vi "RoomAlert.vi"() -> ()   [LabVIEW 2018, in "Visualization.lvlib" / "VisualizeSensor.lvclass"]
doc: "This VI listens for any measurement data associated with the provided PluginName and displays it to the user for analysis. The display is only suitable for data coming from the RoomAlert Plugin."
uses:
  VisualizeSensor.lvclass
  VisualizeBase/VisualizeBase_class/SubVIs/VisualizationOptions.ctl
  <vilib>/Utility/miscctls.llb/LVRectTypeDef.ctl
  Sensor/SensorShared/clSensorData.ctl
  <vilib>/event_ctls.llb/usereventprio.ctl
  VisualizeBase/VisualizeBase_class/Requests/VisUserEventType.ctl
  <extravilib>/ChannelInstances/Tag-bool/Write With Abort.vi
  <extravilib>/ChannelInstances/Tag-bool/Read With Abort.vi
  <extravilib>/ChannelInstances/Tag-bool/Instantiate.vi
  <extravilib>/ChannelInstances/Tag-bool/EndpointRead.vi
  <vilib>/Utility/error.llb/Error Cluster From Error Code.vi
  <extravilib>/ChannelInstances/Tag-bool/Endpoint.vi
  <vilib>/ErrorRing/Error Ring.xnode
  <userlib>/NIST/NISTErrorLib/NISTErrorLib.lvlib
  VisualizeBase/VisualizeBase_class/VisualizeBase.lvclass
  Sensor/SensorShared/SensorShared.lvlib
  Sensor/SensorModule/SensorModule.lvlib
  <extravilib>/ChannelInstances/Tag-bool.lvlib
  TestClass/Test.lvclass
  StatusAndLog/VisualizeStatus.lvclass
  Sensor/SensorPlugins/SensorPlugins.lvlib
panel:
  in  "btnPause":bool=TRUE
  out "VisualizationProperties":T1={"PauseAtStartup"=TRUE, "LogData"=FALSE, "LaunchInSubPanel"=TRUE, "FPMonitor"=0, "FPWindowBounds"={"Left"=0, "Top"=0, "Right"=0, "Bottom"=0}, "MonitorBounds"={"Left"=0, "Top"=0, "Right"=0, "Bottom"=0}}
  in  "INIFilePath":path
  in  "ModuleID":i32
  in  "Log Data":bool=TRUE
  in  "btnStop":bool
  in  "btnReset":bool
  in  "btnClearTest":bool
  in  "btnStopModule":bool
  out "Chart":waveform(dbl)[](graph)=[{"t0"=timestamp(3657200531.6397257 s since 1904-01-01), "dt"=1.0, "Y"=[46.19]}, {"t0"=timestamp(3657200531.6397257 s since 1904-01-01), "dt"=1.0, "Y"=[2.0]}, {"t0"=timestamp(3657200531.6397257 s since 1904-01-01), "dt"=1.0, "Y"=[60.0]}]
  out "LightTower":T3
  out "ErrorArray":errorcluster[](array[cluster])
  out "Incorrect DataType?":bool
  out "String Results":string="Sensor.RoomAlert1"
  in  "PluginName":string="Sensor.RoomAlert1"
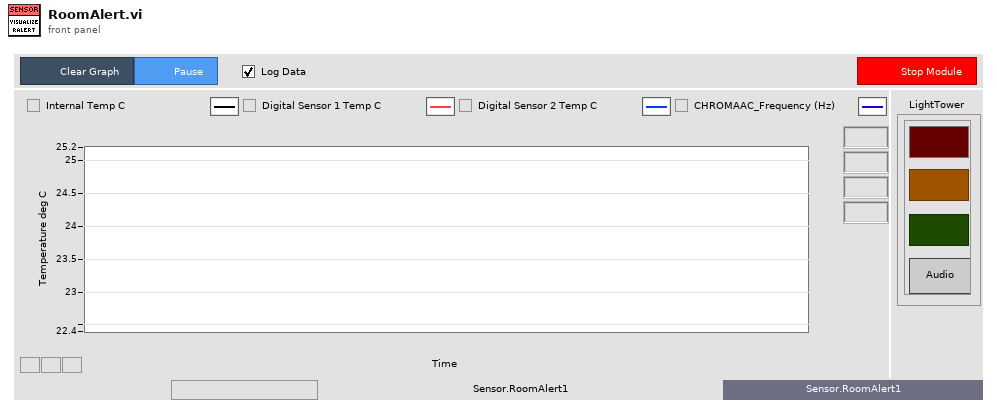
[diagram p1: front panel]
types:
  T1 = typedef "Visualization.lvlib/VisualizeBase.lvclass/VisualizationOptions.ctl" = cluster{"PauseAtStartup":bool, "LogData":bool, "LaunchInSubPanel":bool, "FPMonitor":u16, "FPWindowBounds":T2, "MonitorBounds":cluster{"Left":i16, "Top":i16, "Right":i16, "Bottom":i16}}
  T2 = typedef "LVRectTypeDef.ctl" = cluster{"Left":i16, "Top":i16, "Right":i16, "Bottom":i16}
  T3 = cluster{"Red":bool, "Amber":bool, "Green":bool, "Audio":bool}
  T4 = enum16{"open", "open or create", "create or replace", "create", "open (read-only)"}
  T5 = typedef "Visualization.lvlib/VisualizeBase.lvclass/VisRequestEvents.ctl" = cluster{"StopRequest":refnum<user-event>, "ResetRequest":refnum<user-event>, "FP Pop In or Out":refnum<user-event>}
  T6 = typedef "SensorShared.lvlib/clBroadcastEvents.ctl" = cluster{"DidInit":refnum<user-event>, "StatusUpdate":refnum<user-event>, "ErrorReport":refnum<user-event>, "DidStop":refnum<user-event>, "PathToINI":refnum<user-event>, "SensorReport":refnum<user-event>, "SensorConfig":refnum<user-event>}
  T7 = typedef "SensorShared.lvlib/clSensorData.ctl" = cluster{"SensorType":string, "SensorData":variant}
  T8 = typedef "Visualization.lvlib/VisualizeBase.lvclass/VisUserEventType.ctl" = cluster{"BusIndex":i8, "Data":variant}
  T9 = typedef "usereventprio.ctl" = enum32{"high priority", "normal priority"}
  T10 = cluster{"Red":bool, "Amber":bool, "Green":bool, "Audio":bool}[]
  T11 = typedef "Tag-bool.lvlib/))Channel.ctl" = refnum<queue>
  T12 = typedef "sizeaction.ctl" = enum32{"Minimized", "Maximized", "Resized"}
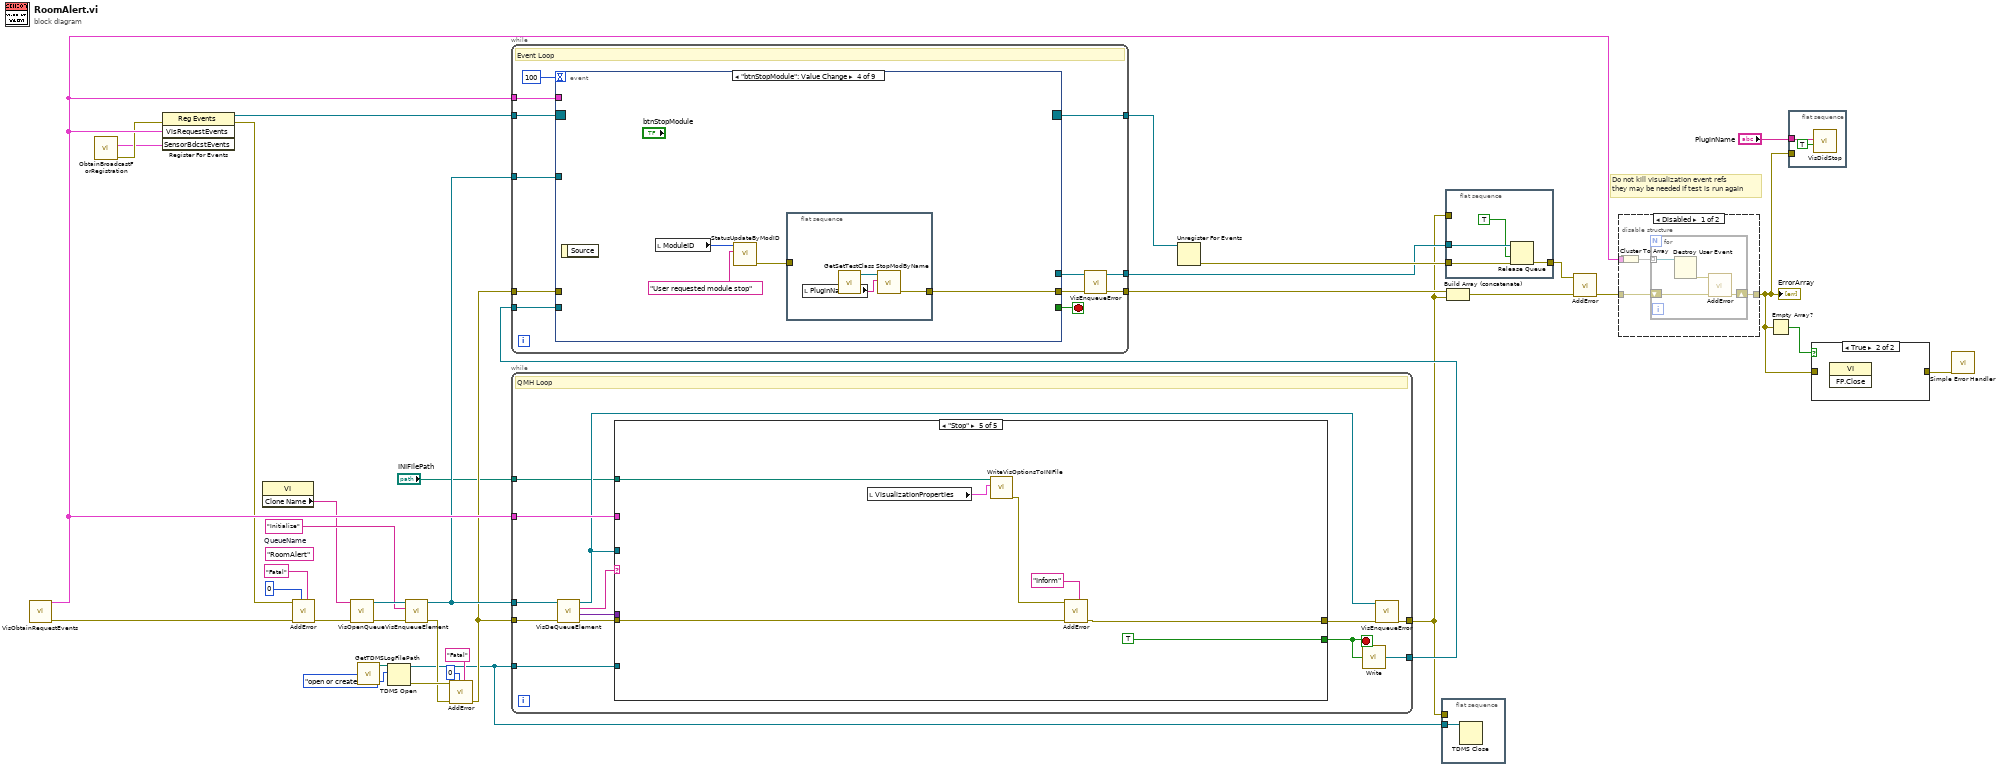
[diagram p0: block diagram]
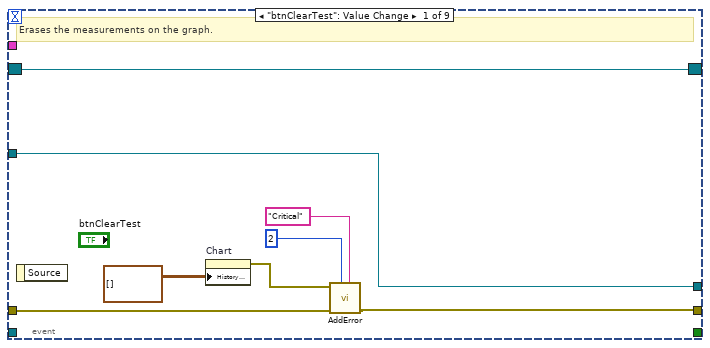
[diagram p3: hidden frame]
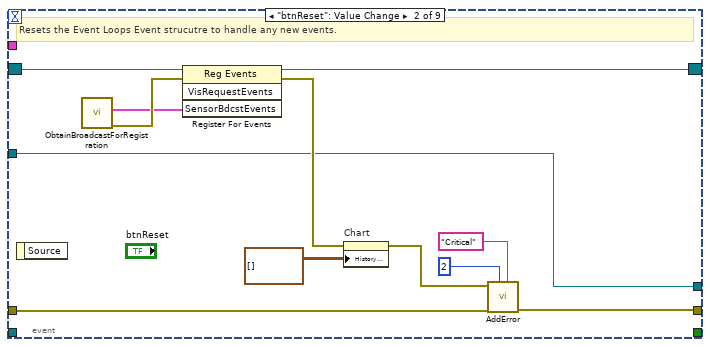
[diagram p4: hidden frame]
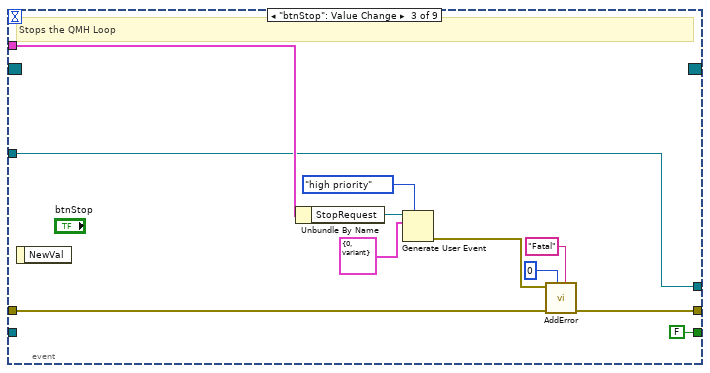
[diagram p5: hidden frame]
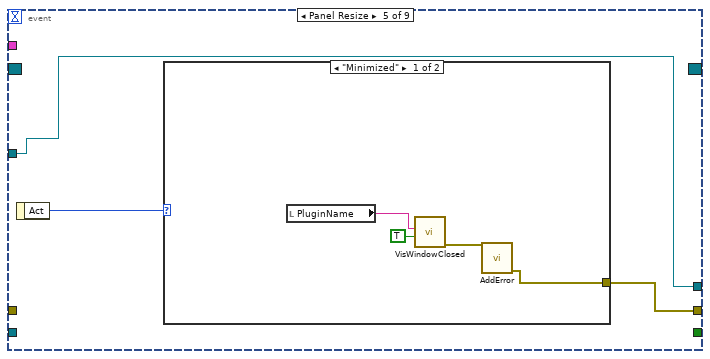
[diagram p6: hidden frame]
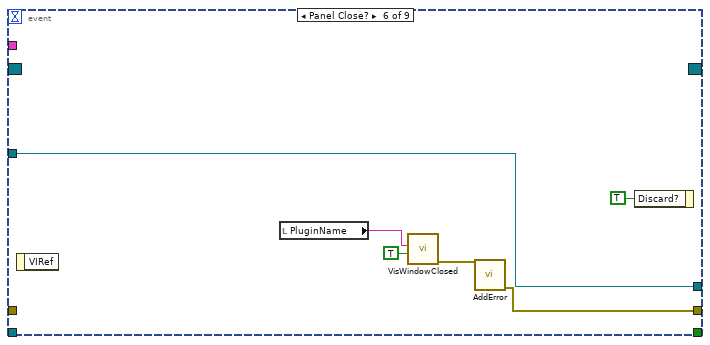
[diagram p8: hidden frame]
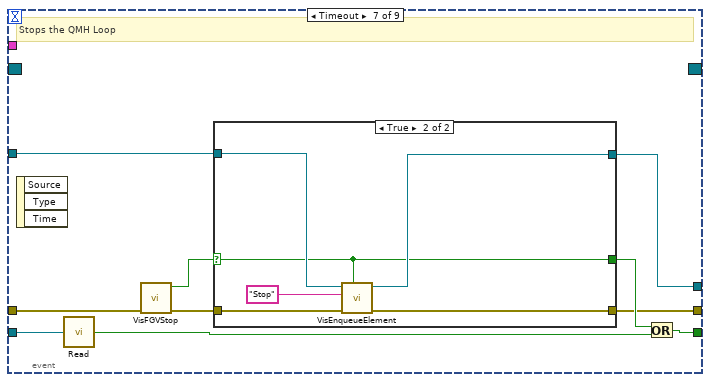
[diagram p9: hidden frame]
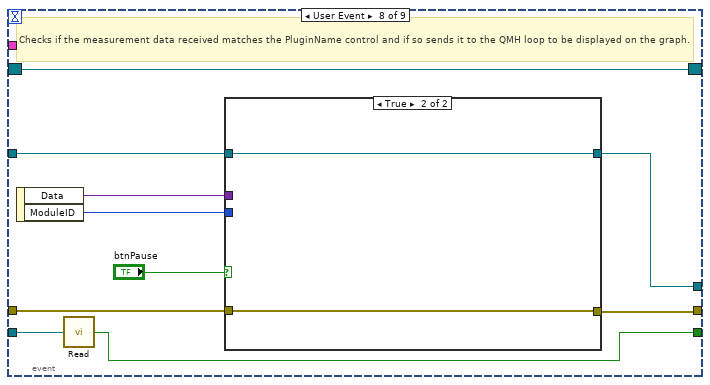
[diagram p11: hidden frame]
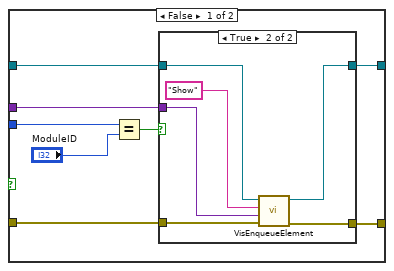
[diagram p12: hidden frame]
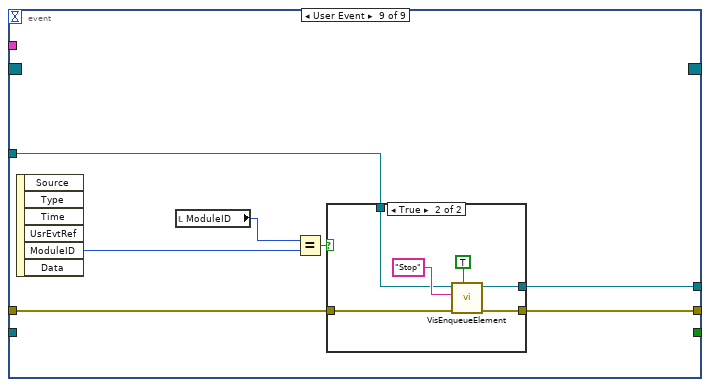
[diagram p14: hidden frame]
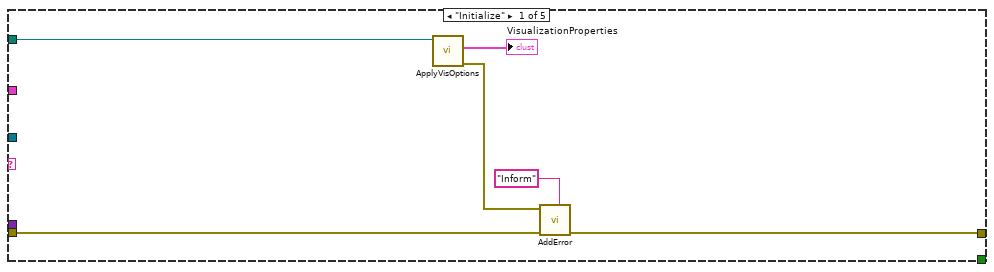
[diagram p16: hidden frame]
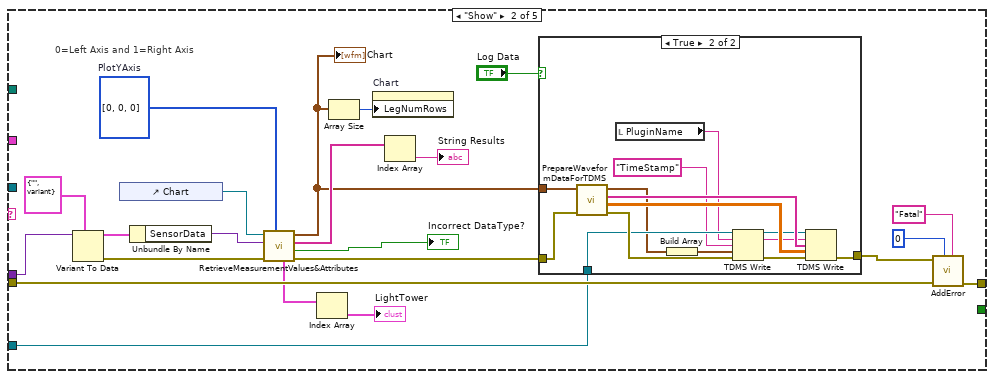
[diagram p17: hidden frame]
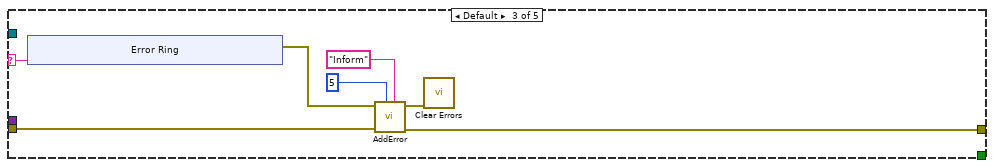
[diagram p19: hidden frame]
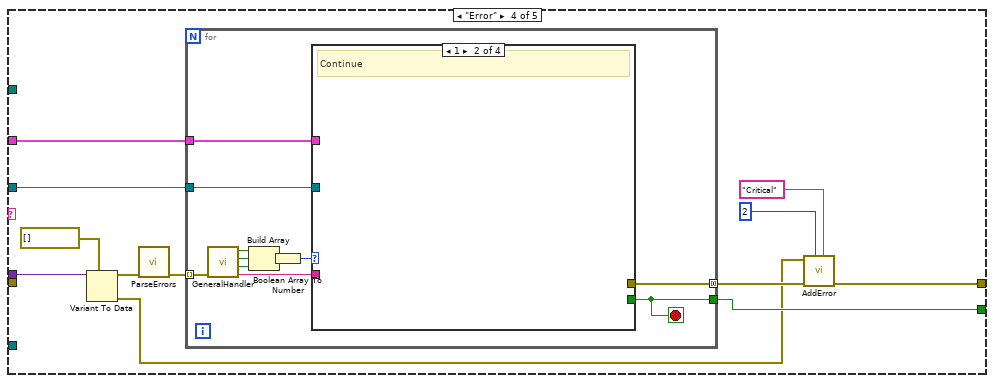
[diagram p20: hidden frame]
diagram:
  (unwired) "RoomAlert"  # QueueName
  # "Do not kill visualization event refs\nthey may be needed if test is run again"
  n1 = call "VisObtainRequestEvents.vi"() -> ("Error"=w27:errorcluster[], "VisRequestEvents"=w29:T5)  [unwired: 10 in]
  n2 = call "ObtainBroadcastForRegistration.vi"() -> ("error out"=w23:errorcluster, "SensorBdcstEvents"=w15:T6)  [unwired: 10 in]
  n3 = register-events(error in=w23, w29, w15) -> (reference out=w36:refnum<event-registration>, error out=w26:errorcluster)  [unwired: 1 in]
  n4 = property class="VI"() -> ("Clone Name"=w13:string)  [unwired: 2 in, 2 out]
  n5 = call <userlib>:"AddError.vi"("Severity"="Fatal", "Priority"=u8 0, "ErrorArray In"=w27, "error in (no error)"=w26) -> ("ErrorArray Out"=w22:errorcluster[])  [unwired: 6 in, 1 out]
  n6 = call "VisOpenQueue.vi"("Error Array In"=w22, "QueueName"=w13) -> ("Error Array Out"=w20:errorcluster[], "queue out"=w21:refnum<queue>)  [unwired: 8 in]
  n7 = call "GetTDMSLogFilePath.vi"() -> ("TDMS Log File Path"=w12:path)  [unwired: 11 in]
  n8 = TDMS Open(10:T4."open or create" ("operation (0:open)"), 11:w12) -> (0:w9:errorcluster, 3:w5:refnum<k34>)  [unwired: 5 in]
  n9 = call "VisEnqueueElement.vi"("Error Array In"=w20, "Message"="Initialize", "queue in"=w21) -> ("Error Array Out"=w8:errorcluster[], "queue out"=w18:refnum<queue>)  [unwired: 7 in]
  n10 = call <userlib>:"AddError.vi"("Severity"="Fatal", "Priority"=u8 0, "ErrorArray In"=w8, "error in (no error)"=w9) -> ("ErrorArray Out"=w7:errorcluster[])  [unwired: 6 in, 1 out]
  n11 = while {
    tunnel: w7 -> [w43]
    tunnel: [w46] -> w4
    tunnel: w18 -> [w42]
    tunnel: w29 -> [w48]
    tunnel: [w39] -> w14
    tunnel: w5 -> [w38]
    tunnel: "INIFilePath" -> [w37]
    stop <- w49 stop-if-true
    # "QMH Loop"
    n12 = call "VisDeQueueElement.vi"("Error Array In"=w43, "Queue In"=w42) -> ("Error Array Out"=w41:errorcluster[], "Data"=w44:variant, "Message"=w45:string, "Queue Out"=w40:refnum<queue>)  [unwired: 6 in]
    n13 = case shown="\"Stop\"" w45 {
      selector: w45 -> [_ _ w99 _ _]
      tunnel: w44 -> [_ w72 _ w118 _]
      tunnel: w41 -> [w52 w75 w97 _ w147]
      tunnel: [w53 w77 w96 w108 w146] -> w47
      tunnel: [_ _ _ w114 TRUE] -> w49
      tunnel: w48 -> [_ _ _ w113 _]
      tunnel: w40 -> [_ _ _ w112 _]
      tunnel: w38 -> [_ w63 _ _ _]
      tunnel: w37 -> [w51 _ _ _ w148]
      frame "Initialize" {
        n14 = call "ApplyVisOptions.vi"("INIFilePath"=w51) -> ("error out"=w55:errorcluster, "VisualizationProperties"=→"VisualizationProperties":T1)  [unwired: 9 in]
        n15 = call <userlib>:"AddError.vi"("Severity"="Inform", "ErrorArray In"=w52, "error in (no error)"=w55) -> ("ErrorArray Out"=w53:errorcluster[])  [unwired: 7 in, 1 out]
      }
      frame "Show" {
        w69 = u32[] [0, 0, 0]  # PlotYAxis
        # "0=Left Axis and 1=Right Axis"
        n16 = Variant To Data(type=T7 {"SensorType"="", "SensorData"=variant} ("clSensorData"), Variant=w72) -> (data=w70:T7, error out=w71:errorcluster)  [unwired: 1 in]
        n17 = control-ref of="Chart"() -> (w76:refnum<vi>)
        n18 = Unbundle By Name(w70) -> ("SensorData"=w67:variant)
        n19 = call "RetrieveMeasurementValues&Attributes.vi"("PlotYScale"=w69, "error in (no error)"=w71, "Variant"=w67, "WaveformChartReference"=w76) -> ("error out"=w66:errorcluster, "Incorrect DataType?"=→"Incorrect DataType?":bool, "Array Of Strings"=w62:string[], "WaveformArrayOut"=w56:waveform(dbl)[], "LightTower"=w60:T10)  [unwired: 3 in]
        "Chart" <- w56
        n20 = Index Array(array=w60) -> (element=→"LightTower":T3)  [unwired: 1 in]
        n21 = Array Size(array=w56) -> (size(s)=w57:i32)
        n22 = property on="Chart" class="WFChart (strict)"("LegNumRows"=w57) -> ()  [unwired: 2 in, 2 out]
        n23 = Index Array(array=w62) -> (element=→"String Results":string)  [unwired: 1 in]
        n24 = case shown="True" "Log Data" {
          tunnel: w66 -> [w78 w91]
          tunnel: [w78 w92] -> w65
          tunnel: w56 -> [_ w90]
          tunnel: w63 -> [_ w85]
          frame False {
          }
          frame True {
            n25 = call "PrepareWaveformDataForTDMS.vi"("error in (no error)"=w91, "WaveformArray in"=w90) -> ("error out"=w89:errorcluster, "Measurement Data"=w87:dbl[][], "Channel Names"=w88:string[], "TimeStamp"=w80:timestamp)  [unwired: 6 in]
            n26 = local read "PluginName"() -> (w83:string)
            n27 = Build Array(w80) -> (w79:timestamp[])
            n28 = TDMS Write(0:w85, 5:w83, 7:"TimeStamp" ("PluginName"), 9:w79, 11:w89) -> (4:w84:refnum<k34>, 6:w82:string, 15:w86:errorcluster)  [unwired: 1 in, 1 out]
            n29 = TDMS Write(0:w84, 5:w82, 7:w88, 9:w87, 11:w86) -> (15:w92:errorcluster)  [unwired: 1 in, 3 out]
          }
        }
        n30 = call <userlib>:"AddError.vi"("Severity"="Fatal" ("String"), "Priority"=u8 0, "ErrorArray In"=w75, "error in (no error)"=w65) -> ("ErrorArray Out"=w77:errorcluster[])  [unwired: 6 in, 1 out]
      }
      frame Default {
        n31 = xnode "Error Ring"("parameter 0"=w99) -> ("error out"=w98:errorcluster)
        n32 = call <userlib>:"AddError.vi"("Severity"="Inform" ("String"), "Priority"=u8 5, "ErrorArray In"=w97, "error in (no error)"=w98) -> ("ErrorArray Out"=w96:errorcluster[], "error out"=w95:errorcluster)  [unwired: 6 in]
        n33 = call <vilib>:"Clear Errors.vi"("error in (no error)"=w95) -> ()  [unwired: 5 in, 2 out]
      }
      frame "Error" {
        n34 = Variant To Data(type=errorcluster[] [], Variant=w118) -> (data=w116:errorcluster[], error out=w107:errorcluster)  [unwired: 1 in]
        n35 = call <userlib>:"ParseErrors.vi"("ErrorArray"=w116) -> ("ErrorArray"=w115:errorcluster[])  [unwired: 8 in, 2 out]
        n36 = for {
          tunnel: w115 -> [w129] mode=indexing
          tunnel: [w123] -> w109 mode=concatenating
          tunnel: [w121] -> w114
          tunnel: w113 -> [w120]
          tunnel: w112 -> [w119]
          stop <- w121 stop-if-true
          n37 = call <userlib>:"GeneralHandler.vi"("error in (no error)"=w129) -> ("Severity"=w122:string, "Stop"=w126:bool, "Abort"=w127:bool, "Continue"=w128:bool)  [unwired: 6 in, 1 out]
          n38 = Build Array(w128, w127, w126) -> (w125:bool[])
          n39 = Boolean Array To Number(Boolean array=w125) -> (number=w124:u32)
          n40 = case shown="1" w124 {
            tunnel: [_ _ w134 w143] -> w123
            tunnel: w122 -> [_ _ _ w136]
            tunnel: [_ _ _ w138] -> w121
            tunnel: w120 -> [_ _ _ w137]
            tunnel: w119 -> [_ _ w130 _]
            frame 0, Default {
              # "No Dialog"
            }
            frame 1 {
              # "Continue"
            }
            frame 2 {
              # "Abort, Flush Queue"
              n41 = Flush Queue(queue=w130) -> (error out=w133:errorcluster)  [unwired: 1 in, 2 out]
              n42 = call <userlib>:"AddError.vi"("Severity"="Critical" ("String"), "Priority"=u8 1, "error in (no error)"=w133) -> ("ErrorArray Out"=w134:errorcluster[])  [unwired: 7 in, 1 out]
            }
            frame 4 {
              # "Stop"
              n43 = Unbundle By Name(w137) -> ("StopRequest"=w144:refnum<user-event>)
              n44 = Equal?(x=w136, y="Fatal" ("x")) -> (x = y?=w138:bool)
              n45 = Generate User Event(priority (normal)=usereventprio."high priority", user event=w144, event data cluster=T8 {"BusIndex"=0, "Data"=variant} ("event data")) -> (error out=w142:errorcluster)  [unwired: 1 in, 1 out]
              n46 = call <userlib>:"AddError.vi"("error in (no error)"=w142) -> ("ErrorArray Out"=w143:errorcluster[], "error out"=w139:errorcluster)  [unwired: 9 in]
              n47 = call <vilib>:"Clear Errors.vi"("error in (no error)"=w139) -> ()  [unwired: 5 in, 2 out]
            }
          }
        }
        n48 = call <userlib>:"AddError.vi"("Severity"="Critical", "Priority"=u8 2, "ErrorArray In"=w109, "error in (no error)"=w107) -> ("ErrorArray Out"=w108:errorcluster[])  [unwired: 6 in, 1 out]
      }
      frame "Stop" {
        n49 = local read "VisualizationProperties"() -> (w145:T1)
        n50 = call "WriteVisOptionsToINIFile.vi"("Visualization Options"=w145, "INIFilePath"=w148) -> ("error out"=w149:errorcluster)  [unwired: 8 in, 1 out]
        n51 = call <userlib>:"AddError.vi"("Severity"="Inform", "ErrorArray In"=w147, "error in (no error)"=w149) -> ("ErrorArray Out"=w146:errorcluster[])  [unwired: 7 in, 1 out]
      }
    }
    n52 = call <extravilib>:"Write.vi"("element"=w49) -> ("channel"=w39:T11)  [unwired: 1 out]
    n53 = call "VisEnqueueError.vi"("Error Array In"=w47, "Queue in"=w40) -> ("Error Array Out"=w46:errorcluster[])  [unwired: 8 in, 1 out]
  }
  n54 = while {
    tunnel: w36 -> [w163]
    tunnel: [w157] -> w34
    tunnel: [w161] -> w35
    tunnel: w29 -> [w160]
    tunnel: w7 -> [w159]
    tunnel: w18 -> [w158]
    tunnel: [w154] -> w17
    tunnel: w14 -> [w152]
    stop <- w162 stop-if-true
    # "Event Loop"
    n55 = event shown="[3] \"btnStopModule\": Value Change" {
      selector: w163 -> [w165 w183 _ _ _ _ _ w239 _]
      dyn-events: [w165 w182 _ _ _ _ _ w239 _] -> w161
      timeout: 100 -> [_ _ _ _ _ _ _ _ _]
      tunnel: [_ _ FALSE ("Priority? (F)") _ _ _ w215 w236 _] -> w162
      tunnel: [w168 w180 w187 w198 w203 w210 w217 w241 w265] -> w156
      tunnel: w160 -> [_ _ w186 _ _ _ _ _ _]
      tunnel: w159 -> [w169 w181 w194 _ _ _ w220 w242 w264]
      tunnel: w158 -> [w164 w173 w184 _ w202 w209 w219 w243 w267]
      tunnel: [w164 w173 w184 _ w202 w209 w218 w240 w266] -> w155
      tunnel: w152 -> [_ _ _ _ _ _ w224 w237 _]
      event "btnClearTest": Value Change {
        # "Erases the measurements on the graph."
        n56 = event-data() -> ()  [unwired: 1 in, 1 out]
        n57 = property on="Chart" class="WFChart (strict)"("History Data"=waveform(dbl)[][] []) -> (error out=w167:errorcluster)  [unwired: 2 in, 1 out]
        n58 = call <userlib>:"AddError.vi"("Severity"="Critical", "Priority"=u8 2, "ErrorArray In"=w169, "error in (no error)"=w167) -> ("ErrorArray Out"=w168:errorcluster[])  [unwired: 6 in, 1 out]
      }
      event "btnReset": Value Change {
        # "Resets the Event Loops Event strucutre to handle any new events."
        n59 = event-data() -> ()  [unwired: 1 in, 1 out]
        n60 = call "ObtainBroadcastForRegistration.vi"() -> ("error out"=w174:errorcluster, "SensorBdcstEvents"=w172:T6)  [unwired: 10 in]
        n61 = register-events(reference=w183, error in=w174, w172) -> (reference out=w182:refnum<event-registration>, error out=w176:errorcluster)  [unwired: 1 in]
        n62 = property on="Chart" class="WFChart (strict)"(error in=w176, "History Data"=waveform(dbl)[][] []) -> (error out=w175:errorcluster)  [unwired: 1 in, 1 out]
        n63 = call <userlib>:"AddError.vi"("Severity"="Critical", "Priority"=u8 2, "ErrorArray In"=w181, "error in (no error)"=w175) -> ("ErrorArray Out"=w180:errorcluster[])  [unwired: 6 in, 1 out]
      }
      event "btnStop": Value Change {
        # "Stops the QMH Loop"
        n64 = event-data() -> ()  [unwired: 1 in, 1 out]
        n65 = Unbundle By Name(w186) -> ("StopRequest"=w192:refnum<user-event>)
        n66 = Generate User Event(priority (normal)=usereventprio."high priority", user event=w192, event data cluster=T8 {"BusIndex"=0, "Data"=variant} ("event data")) -> (error out=w193:errorcluster)  [unwired: 1 in, 1 out]
        n67 = call <userlib>:"AddError.vi"("Severity"="Fatal" ("String"), "Priority"=u8 0, "ErrorArray In"=w194, "error in (no error)"=w193) -> ("ErrorArray Out"=w187:errorcluster[])  [unwired: 6 in, 1 out]
      }
      event "btnStopModule": Value Change {
        n68 = event-data() -> ()  [unwired: 1 in, 1 out]
        n69 = local read "ModuleID"() -> (w197:i32)
        n70 = call "StatusUpdateByModID.vi"("Status"="User requested module stop", "Accessors:Module ID"=w197) -> ("error out"=w196:errorcluster)  [unwired: 9 in]
        n71 = flat-sequence {
          tunnel: [w200] -> w198
          tunnel: w196 -> [_]
          frame #0 {
            n72 = local read "PluginName"() -> (w199:string)
            n73 = call "GetSetTestClass.vi"() -> ("Test.lvclass"=w201:refnum<class "Test.lvclass">)  [unwired: 11 in]
            n74 = call "StopModByName.vi"("Module Name"=w199, "Test.lvclass"=w201) -> ("ErrorArray Out"=w200:errorcluster[])  [unwired: 5 in, 4 out]
          }
        }
      }
      event Panel Resize {
        n75 = event-data() -> ("Act"=w204:T12)  [unwired: 1 in]
        n76 = case shown="\"Minimized\"" w204 {
          tunnel: [w205 _] -> w203
          frame "Minimized" {
            n77 = local read "PluginName"() -> (w207:string)
            n78 = call "VisWindowClosed.vi"("Window Closed?"=TRUE ("Window Minimized or Clozed?"), "Module Name"=w207) -> ("error out"=w208:errorcluster)  [unwired: 9 in]
            n79 = call <userlib>:"AddError.vi"("error in (no error)"=w208) -> ("ErrorArray Out"=w205:errorcluster[])  [unwired: 9 in, 1 out]
          }
          frame "Maximized", Default {
          }
        }
      }
      event Panel Close? {
        n80 = event-data() -> ()  [unwired: 1 in, 1 out]
        n81 = local read "PluginName"() -> (w211:string)
        n82 = call "VisWindowClosed.vi"("Window Closed?"=TRUE ("Window Minimized or Clozed?"), "Module Name"=w211) -> ("error out"=w212:errorcluster)  [unwired: 9 in]
        n83 = call <userlib>:"AddError.vi"("error in (no error)"=w212) -> ("ErrorArray Out"=w210:errorcluster[])  [unwired: 9 in, 1 out]
        n84 = event-data("Discard?"=TRUE) -> ()  [unwired: 1 in, 1 out]
      }
      event Timeout {
        # "Stops the QMH Loop"
        n85 = event-data() -> ()  [unwired: 1 in, 3 out]
        n86 = call <extravilib>:"Read.vi"("channel"=w224) -> ("element"=w216:bool)  [unwired: 1 in, 1 out]
        n87 = call "VisFGVStop.vi"("Error In"=w220) -> ("Error Out"=w222:errorcluster[], "Value"=w223:bool)  [unwired: 9 in]
        n88 = case shown="True" w223 {
          selector: w223 -> [w225 w228]
          tunnel: [w227 w231] -> w217
          tunnel: w222 -> [w227 w232]
          tunnel: w219 -> [w226 w230]
          tunnel: [w226 w229] -> w218
          tunnel: [w225 w228] -> w221
          frame False {
          }
          frame True {
            n89 = call "VisEnqueueElement.vi"("Priority? (F)"=w228, "Error Array In"=w232, "Message"="Stop", "queue in"=w230) -> ("Error Array Out"=w231:errorcluster[], "queue out"=w229:refnum<queue>)  [unwired: 6 in]
          }
        }
        n90 = Or(x=w221, y=w216) -> (x .or. y?=w215:bool)
      }
      event User Event {
        # "Checks if the measurement data received matches the PluginName control and if so sends it to the QMH loop to be displayed on the graph."
        n91 = event-data() -> ("Data"=w238:variant, "ModuleID"=w235:i32)  [unwired: 1 in]
        n92 = call <extravilib>:"Read.vi"("channel"=w237) -> ("element"=w236:bool)  [unwired: 1 in, 1 out]
        n93 = case shown="True" "btnPause" {
          tunnel: w243 -> [w251 w261]
          tunnel: w242 -> [w250 w260]
          tunnel: [w249 w260] -> w241
          tunnel: [w248 w261] -> w240
          tunnel: w238 -> [w247 _]
          tunnel: w235 -> [w244 _]
          frame False {
            n94 = Equal?(x=w244, y="ModuleID") -> (x = y?=w246:bool)
            n95 = case shown="True" w246 {
              tunnel: [w252 w258] -> w249
              tunnel: w251 -> [w253 w257]
              tunnel: w250 -> [w252 w259]
              tunnel: [w253 w255] -> w248
              tunnel: w247 -> [_ w256]
              frame False {
              }
              frame True {
                n96 = call "VisEnqueueElement.vi"("Error Array In"=w259, "Data"=w256, "Message"="Show", "queue in"=w257) -> ("Error Array Out"=w258:errorcluster[], "queue out"=w255:refnum<queue>)  [unwired: 6 in]
              }
            }
          }
          frame True {
          }
        }
      }
      event User Event {
        n97 = event-data() -> ("ModuleID"=w263:i32)  [unwired: 1 in, 5 out]
        n98 = local read "ModuleID"() -> (w262:i32)
        n99 = Equal?(x=w262, y=w263) -> (x = y?=w268:bool)
        n100 = case shown="True" w268 {
          tunnel: [w269 w274] -> w265
          tunnel: [w270 w273] -> w266
          tunnel: w267 -> [w270 w272]
          tunnel: w264 -> [w269 w271]
          frame False {
          }
          frame True {
            n101 = call "VisEnqueueElement.vi"("Priority? (F)"=TRUE, "Error Array In"=w271, "Message"="Stop", "queue in"=w272) -> ("Error Array Out"=w274:errorcluster[], "queue out"=w273:refnum<queue>)  [unwired: 6 in]
          }
        }
      }
    }
    n102 = call "VisEnqueueError.vi"("Error Array In"=w156, "Queue in"=w155) -> ("Error Array Out"=w157:errorcluster[], "Queue out"=w154:refnum<queue>)  [unwired: 8 in]
  }
  n103 = Unregister For Events(event registration refnum=w35) -> (error out=w33:errorcluster)  [unwired: 1 in]
  n104 = flat-sequence {
    tunnel: w5 -> [w277]
    tunnel: w4 -> [_]
    frame #0 {
      n105 = TDMS Close(11:w277) -> ()  [unwired: 1 in, 2 out]
    }
  }
  n106 = flat-sequence {
    tunnel: w33 -> [w281]
    tunnel: [w280] -> w31
    tunnel: w17 -> [w279]
    tunnel: w4 -> [_]
    frame #0 {
      n107 = Release Queue(queue=w279, force destroy? (F)=TRUE, error in (no error)=w281) -> (error out=w280:errorcluster)  [unwired: 2 out]
    }
  }
  n108 = Build Array (concatenate)(w34, w4) -> (w32:errorcluster[])
  n109 = call <userlib>:"AddError.vi"("ErrorArray In"=w32, "error in (no error)"=w31) -> ("ErrorArray Out"=w30:errorcluster[])  [unwired: 8 in, 1 out]
  n110 = disable-structure shown="Disabled" {
    disable-tunnel: w30 -> [w284 w290]
    disable-tunnel: w29 -> [w283 _]
    disable-tunnel: [w282 w290] -> w1
    frame Disabled {
      n111 = Cluster To Array(cluster=w283) -> (array=w285:refnum<user-event>[])
      n112 = for {
        tunnel: w285 -> [w289] mode=indexing
        shift-right: [w288] -> w282
        shift-left: w284 -> [w287]
        n113 = Destroy User Event(user event=w289) -> (error out=w286:errorcluster)  [unwired: 1 in]
        n114 = call <userlib>:"AddError.vi"("ErrorArray In"=w287, "error in (no error)"=w286) -> ("ErrorArray Out"=w288:errorcluster[])  [unwired: 8 in, 1 out]
      }
    }
    frame Enabled {
    }
  }
  "ErrorArray" <- w1
  n115 = Empty Array?(array=w1) -> (empty?=w28:bool)
  n116 = flat-sequence {
    tunnel: "PluginName" -> [w292]
    tunnel: w1 -> [_]
    frame #0 {
      n117 = call "VisDidStop.vi"("DidStop?"=TRUE, "Module Name"=w292) -> ()  [unwired: 9 in, 1 out]
    }
  }
  n118 = case shown="True" w28 {
    tunnel: [w293 _] -> w16
    tunnel: w1 -> [w294 _]
    frame False {
      n119 = Merge Errors(w294) -> (w293:errorcluster)
    }
    frame True {
      n120 = invoke class="VI" method="FP.Close"() -> ()  [unwired: 3 in, 3 out]
    }
  }
  n121 = call <vilib>:"Simple Error Handler.vi"("error in (no error)"=w16) -> ()  [unwired: 4 in, 5 out]
